vi "Read_Stream_Data.vi"(8 "error in (no error)":errorcluster, 11 "Refnum in":refnum<k21>) -> (0 "error out":errorcluster, 1 "Desired Position":dbl[](array[numeric]), 2 "Reset to zero position?":bool, 3 "Refnum out":refnum<k21>, 5 "Enabled motor?":bool[](array[boolean]))   [LabVIEW 2015]
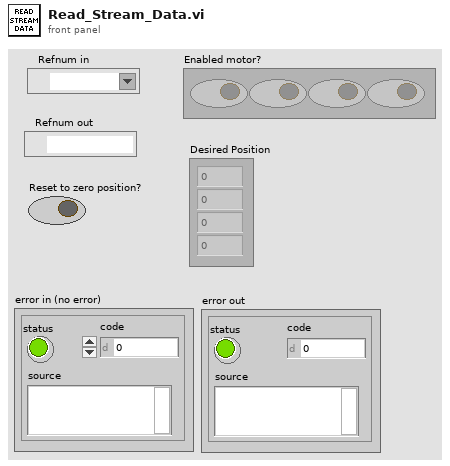
[diagram p1: front panel]
types:
  T1 = cluster{"Desired Position":u16, "Enable?":bool, "Reset?":bool}[]
  T2 = cluster{"Desired Position":u16, "Enable?":bool, "Reset?":bool}
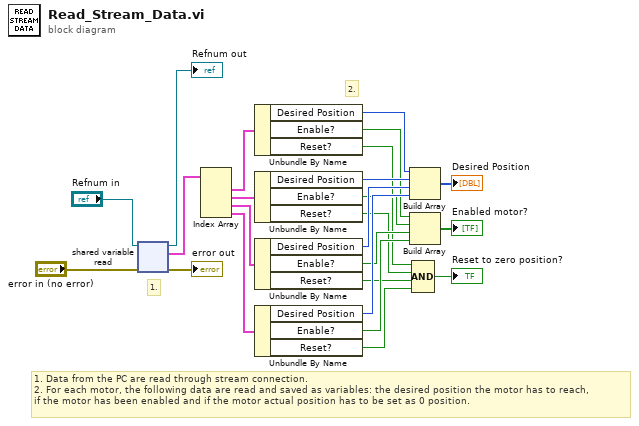
[diagram p0: block diagram]
diagram:
  # "2."
  # "1."
  # "1. Data from the PC are read through stream connection.\n2. For each motor, the following data are read and saved as variables: the desired position the motor has to reach,\nif the motor has been enabled and if the motor actual position has to be set as 0 position."
  n1 = shared-variable-read("Refnum in", "error in (no error)") -> (→"Refnum out":refnum<k21>, →"error out":errorcluster, w5:T1)  [unwired: 1 in, 1 out]
  n2 = Index Array(array=w5) -> (element #1=w6:T2, element #2=w7:T2, element #3=w8:T2, element #4=w9:T2)  [unwired: 4 in]
  n3 = Unbundle By Name(w6) -> ("Desired Position"=w20:u16, "Enable?"=w15:bool, "Reset?"=w10:bool)
  n4 = Unbundle By Name(w7) -> ("Desired Position"=w21:u16, "Enable?"=w16:bool, "Reset?"=w11:bool)
  n5 = Unbundle By Name(w8) -> ("Desired Position"=w22:u16, "Enable?"=w17:bool, "Reset?"=w13:bool)
  n6 = Unbundle By Name(w9) -> ("Desired Position"=w23:u16, "Enable?"=w18:bool, "Reset?"=w14:bool)
  n7 = Build Array(w20, w21, w22, w23) -> (→"Desired Position":u16[])
  n8 = Build Array(w15, w16, w17, w18) -> (→"Enabled motor?":bool[])
  n9 = Compound Arithmetic op=AND(w10, w11, w13, w14) -> (→"Reset to zero position?":bool)
